vi "Untitled 1.vi"() -> ()   [LabVIEW 2019]
panel:
  out "sampling info":cluster{"Fs":dbl, "#s":dbl}={"Fs"=1000.0, "#s"=1000.0}
  out "offset":dbl
  out "square wave duty cycle (%)":dbl=50.0
  out "phase":dbl
  out "amplitude":dbl=1.0
  out "frequency":dbl=10.0
  out "signal type":T1(ring)
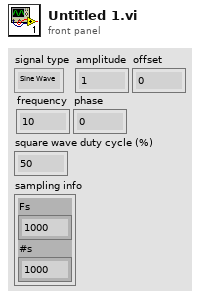
[diagram p1: front panel]
types:
  T1 = enum16{"Sine Wave", "Triangle Wave", "Square Wave", "Sawtooth Wave"}
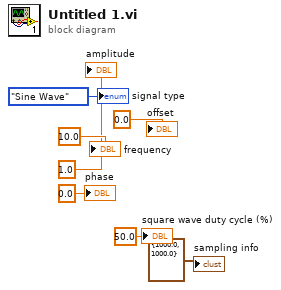
[diagram p0: block diagram]
diagram:
  "signal type" <- T1."Sine Wave" ("signal type")
  "frequency" <- 10.0 ("frequency")
  "amplitude" <- 1.0 ("amplitude")
  "phase" <- 0.0 ("phase")
  "square wave duty cycle (%)" <- 50.0 ("square wave duty cycle (%)")
  "offset" <- 0.0 ("offset")
  "sampling info" <- cluster{"Fs":dbl, "#s":dbl} {"Fs"=1000.0, "#s"=1000.0} ("sampling info")
